vi "Set Payload File Path.vi"(8 "error in":errorcluster, 10 "frame array file path":path, 11 "custom device ref in":T1 format="%.0x") -> (0 "error out":errorcluster, 3 "custom device ref out out":T1 format="%.0x")   [LabVIEW 2020, in "AIM ARINC 664 Scripting.lvlib"]
uses:
  AIM ARINC 664 Scripting.lvlib
  Constants.vi
  <vilib>/NI VeriStand/Custom Device API/Custom Device API.lvlib
  <vilib>/NI VeriStand/Custom Device Tools/Custom Device Utility Library/Custom Device Utility Library.lvlib
  <vilib>/NI VeriStand/Custom Device Tools/Custom Device Utility Library/NI VeriStand - Search for Item by GUID.vi
  <vilib>/NI VeriStand/Custom Device API/Set Item Property (Dependent File).vi
  <vilib>/NI VeriStand/Custom Device API/Custom Device Item Ref.ctl
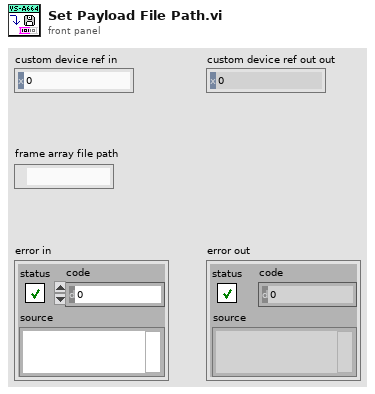
[diagram p1: front panel]
types:
  T1 = typedef "Custom Device API.lvlib/Custom Device Item Ref.ctl" = u64
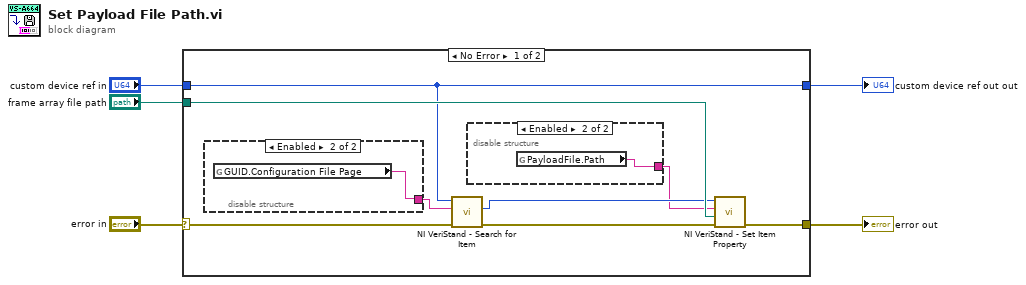
[diagram p0: block diagram]
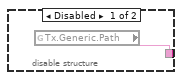
[diagram p2: hidden frame]
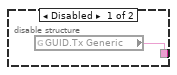
[diagram p3: hidden frame]
diagram:
  n1 = case shown="No Error" "error in" {
    selector: "error in" -> [w12 w19]
    tunnel: "custom device ref in" -> [w9 w18]
    tunnel: [w13 w19] -> w4
    tunnel: [w9 w18] -> w3
    tunnel: "frame array file path" -> [w11 _]
    frame No Error {
      n2 = disable-structure shown="Enabled" {
        disable-tunnel: [w16 w17] -> w7
        frame Disabled {
          n3 = global read "Constants.vi" "GUID.Tx Generic"() -> (w16:string)
        }
        frame Enabled {
          n4 = global read "Constants.vi" "GUID.Configuration File Page"() -> (w17:string)
        }
      }
      n5 = call-poly <vilib>:"NI VeriStand - Search for Item.vi"("error in"=w12, "Item GUID"=w7, "Section Ref in"=w9) -> ("error out"=w10:errorcluster, "Item Ref"=w8:T1)  [unwired: 5 in, 2 out]
      n6 = disable-structure shown="Enabled" {
        disable-tunnel: [w14 w15] -> w6
        frame Disabled {
          n7 = global read "Constants.vi" "Tx.Generic.Path"() -> (w14:string)
        }
        frame Enabled {
          n8 = global read "Constants.vi" "PayloadFile.Path"() -> (w15:string)
        }
      }
      n9 = call-poly <vilib>:"NI VeriStand - Set Item Property.vi"("error in (no error)"=w10, "Path"=w11, "Property Name"=w6, "Item Ref in"=w8) -> ("error out"=w13:errorcluster)  [unwired: 5 in, 2 out]
    }
    frame Error {
    }
  }
  "error out" <- w4
  "custom device ref out out" <- w3
